vi "Sim Stripped..vi"() -> ()   [LabVIEW 2013]
doc: "This is the FPGA VI for the 10-Tap 8-Bit Camera with DRAM example. This example demonstrates how to acquire images from a 10-tap, 8-bit, extended configuration, Camera Link camera and transfer the images to the host. This example supports area scan and line scan cameras for both continuous and finite acquisitions.\n\nThis example also demonstrates the use of DRAM as a frame buffer for very high speed acquisitions. Data packing and flow-control are also employed to maximize use of the available DRAM and FIFOs in terms of both memory space and performance.\n\nAdditionally, the example demonstrates the serial server, which allows third-party camera configuration utilities to communicate with the camera using the Camera Link serial interface while this VI is running."
uses:
  <vilib>/rvi/DataTransferAndStorage/Container/XNode/niFpgaContainer.xnode
  <vilib>/Platform/TimedLoop/XDataNode/XDataNode.xnode
  <vilib>/Platform/TimedLoop/XDataNode/timing_clust.ctl
  <vilib>/Platform/TimedLoop/XDataNode/XDNodeRunTimeDep.lvlib
  <vilib>/Platform/TimedLoop/XDataNode/wakeup.ctl
  <vilib>/Platform/TimedLoop/XDataNode/nitl_modes.ctl
  <vilib>/eio/EIONode/EIONode.xnode
  <vilib>/rvi/eio/common/nirviEmuTemplateMethod_errors.vi
  <vilib>/rvi/FIFO/Fifo_Resource/nirvififoEmulationGetNumberOfElementsToRead.vi
  <vilib>/rvi/interface/RandomDataEmulation/nirviRandomDataFpgaReadWriteTemplate.vi
  <vilib>/rvi/FIFO/Fifo_Resource/nirvififoEmulationRead.vi
  <vilib>/rvi/FIFO/Fifo_Resource/nirvififoEmulationWrite.vi
  Common/CL Data to Pixels/10 Tap 8-Bit.vi
  FPGA/10-Tap Data/10-Tap Conversion Enum.ctl
  FPGA/Globals/Accumulated Sector Intensity.vi
  FPGA/Globals/Pixel Location Global.vi
  FPGA/Globals/Wing Square Wave Frequency Global.vi
  <vilib>/rvi/FIFO/Fifo_Resource/nirvififoEmulationGetNumberOfElementsToWrite.vi
  FPGA/Globals/Sector Parameter Global.vi
  Common/CL Signal Mapping.ctl
  Common/CL Configuration.ctl
  FPGA/Sector/Accumulate/Sector Parameter Cluster.ctl
panel:
  in  "[Average BG Intensity]":u8[](array[numeric])=[0, 0, 0, 0, 0, 0, 0, 0, 0, 0, 0, 0, 0, 0, 0, 0, 0, 0, 0, 0, 0, 0, 0, 0, 0, 0, 0, 0, 0, 0, 0, 0]
  in  "Sector Threshold":u8
  in  "# of Frames to Average":u8
  in  "Sector Parameters Right":T1={"Start Angle"=0.13543701171875, "End Angle"=0.30462646484375, "Inner Radius"=309, "Outter Radius"=405, "Hinge X"=1106, "Hinge Y"=803, "NumWingSectors"=8}
  in  "Sector Parameters Left":T1={"Start Angle"=0.6541748046875, "End Angle"=0.856201171875, "Inner Radius"=309, "Outter Radius"=405, "Hinge X"=947, "Hinge Y"=829, "NumWingSectors"=8}
  in  "CL Config.Configuration":T2=enum."Full"
  in  "CL Config.Signal Mapping":T3=enum."Basler 10-tap"
  in  "CL Config.Line Scan":bool
  in  "CL Config.DVAL Active High":bool=TRUE
  in  "CL Config.LVAL Active High":bool=TRUE
  in  "CL Config.FVAL Active High":bool=TRUE
  in  "CL Config.Spare Active High":bool=TRUE
  in  "Acq Control.Line Scan Height":u32
  in  "Acq Control.Frames To Acq":u32
  in  "Acq Control.Acquire":bool
  in  "Acq Control.Cancel Acq":bool
  in  "Acq Control.Ignore DVAL":bool
  in  "Acq Control.Initialize":bool
  out "Acq Status.Acq In Progress":bool
  out "Acq Status.Clocks Per Line":u32
  out "Acq Status.Frames Acq'd":u32
  out "Acq Status.Lines Per Frame":u32
  out "Acq Status.DMA Write Timeout":bool
  out "Acq Status.Initialized":bool
  in  "UART.Baud Rate":u8
  in  "UART.Transmit":bool
  in  "UART.Tx Data":u8[](array[numeric])=[0, 0, 0, 0, 0, 0, 0, 0, 0, 0] format="%02x"
  in  "UART.Set Baud Rate":bool
  in  "UART.Byte Mode":bool=TRUE
  out "UART.Rx Ready":bool
  out "UART.Break Indicator":bool
  out "UART.Framing Error":bool
  out "UART.Overrun Error":bool
  out "UART.Tx Ready":bool
  out "UART.Rx Data":u8 format="%02x"
  in  "UART.Receive":bool
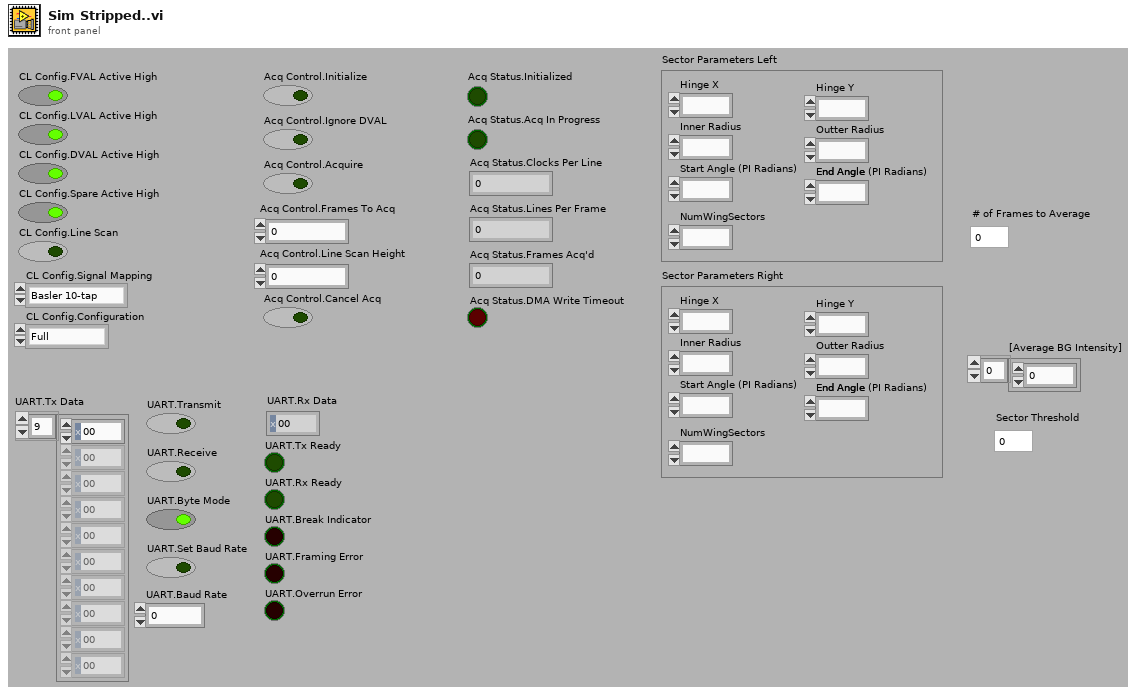
[diagram p1: front panel]
types:
  T1 = typedef "Sector Parameter Cluster.ctl" = cluster{"Start Angle":fxp<+/-,17,2>, "End Angle":fxp<+,17,3>, "Inner Radius":u16, "Outter Radius":u16, "Hinge X":u16, "Hinge Y":u16, "NumWingSectors":u8}
  T2 = typedef "CL Configuration.ctl" = enum8{"Base", "Medium", "Full"}
  T3 = typedef "CL Signal Mapping.ctl" = enum8{"Standard", "Basler 10-tap", "Vosskühler 10-tap"}
  T4 = typedef "XDNodeRunTimeDep.lvlib/timing_clust.ctl" = cluster{"Expected End [f-1]":u64, "Actual End [f-1]":u64, "Finished Late? [f-1]":bool, "Expected End [i-1]":u64, "Actual End [i-1]":u64, "Finished Late? [i-1]":bool, "Expected Start [i]":u64, "Actual Start [i]":u64, "Expected Start [f]":u64, "Actual Start [f]":u64, "Source Name":string, "Structure Name":string, "Period":i64, "Deadline":i64, "Offset":i64, "Start":i64, "Priority":i32, "Timeout":i32, "Mode":T5, "Wakeup Reason":T6, "Error":errorcluster, "Source Type":string, "Secondary Source Type":string, "Global End Time":u64, "Global Start Time":u64, "Frame Duration":u64, "Iteration Duration":u64, "Assigned CPU":i32, "I/O Scan Engine Mode":u32}
  T5 = typedef "XDNodeRunTimeDep.lvlib/nitl_modes.ctl" = enum32{"No Change", "Process missed periods, maintain original phase", "Discard missed periods, maintain original phase", "Process missed periods, ignore original phase", "Discard missed periods, ignore original phase"}
  T6 = typedef "XDNodeRunTimeDep.lvlib/wakeup.ctl" = enum32{"Normal", "Aborted", "Asynchronous wakeup", "Timing source error", "Timed loop error", "Timeout"}
  T7 = typedef "10-Tap Conversion Enum.ctl" = enum16{"10-Tap to 16 and 64", "16 and 64 to 10-Tap"}
  T8 = cluster{"Enables Valid":bool, "Frame Valid":bool, "Line Valid":bool, "Data Valid":bool}
  T9 = typedef "10-Tap 8-bit Cluster.ctl" = cluster{"Pixel 0":u8, "Pixel 1":u8, "Pixel 2":u8, "Pixel 3":u8, "Pixel 4":u8, "Pixel 5":u8, "Pixel 6":u8, "Pixel 7":u8, "Pixel 8":u8, "Pixel 9":u8}
  T10 = cluster{"Tx Data":u8[], "Transmit":bool, "Receive":bool, "Byte Mode":bool, "Set Baud Rate":bool, "Baud Rate":u8}
  T11 = cluster{"Rx Data":u8, "Turn Off Transmit":bool, "Turn Off Receive":bool, "Turn Off Set Baud Rate":bool, "Tx Ready":bool, "Rx Ready":bool, "Break Indicator":bool, "Framing Error":bool, "Overrun Error":bool}
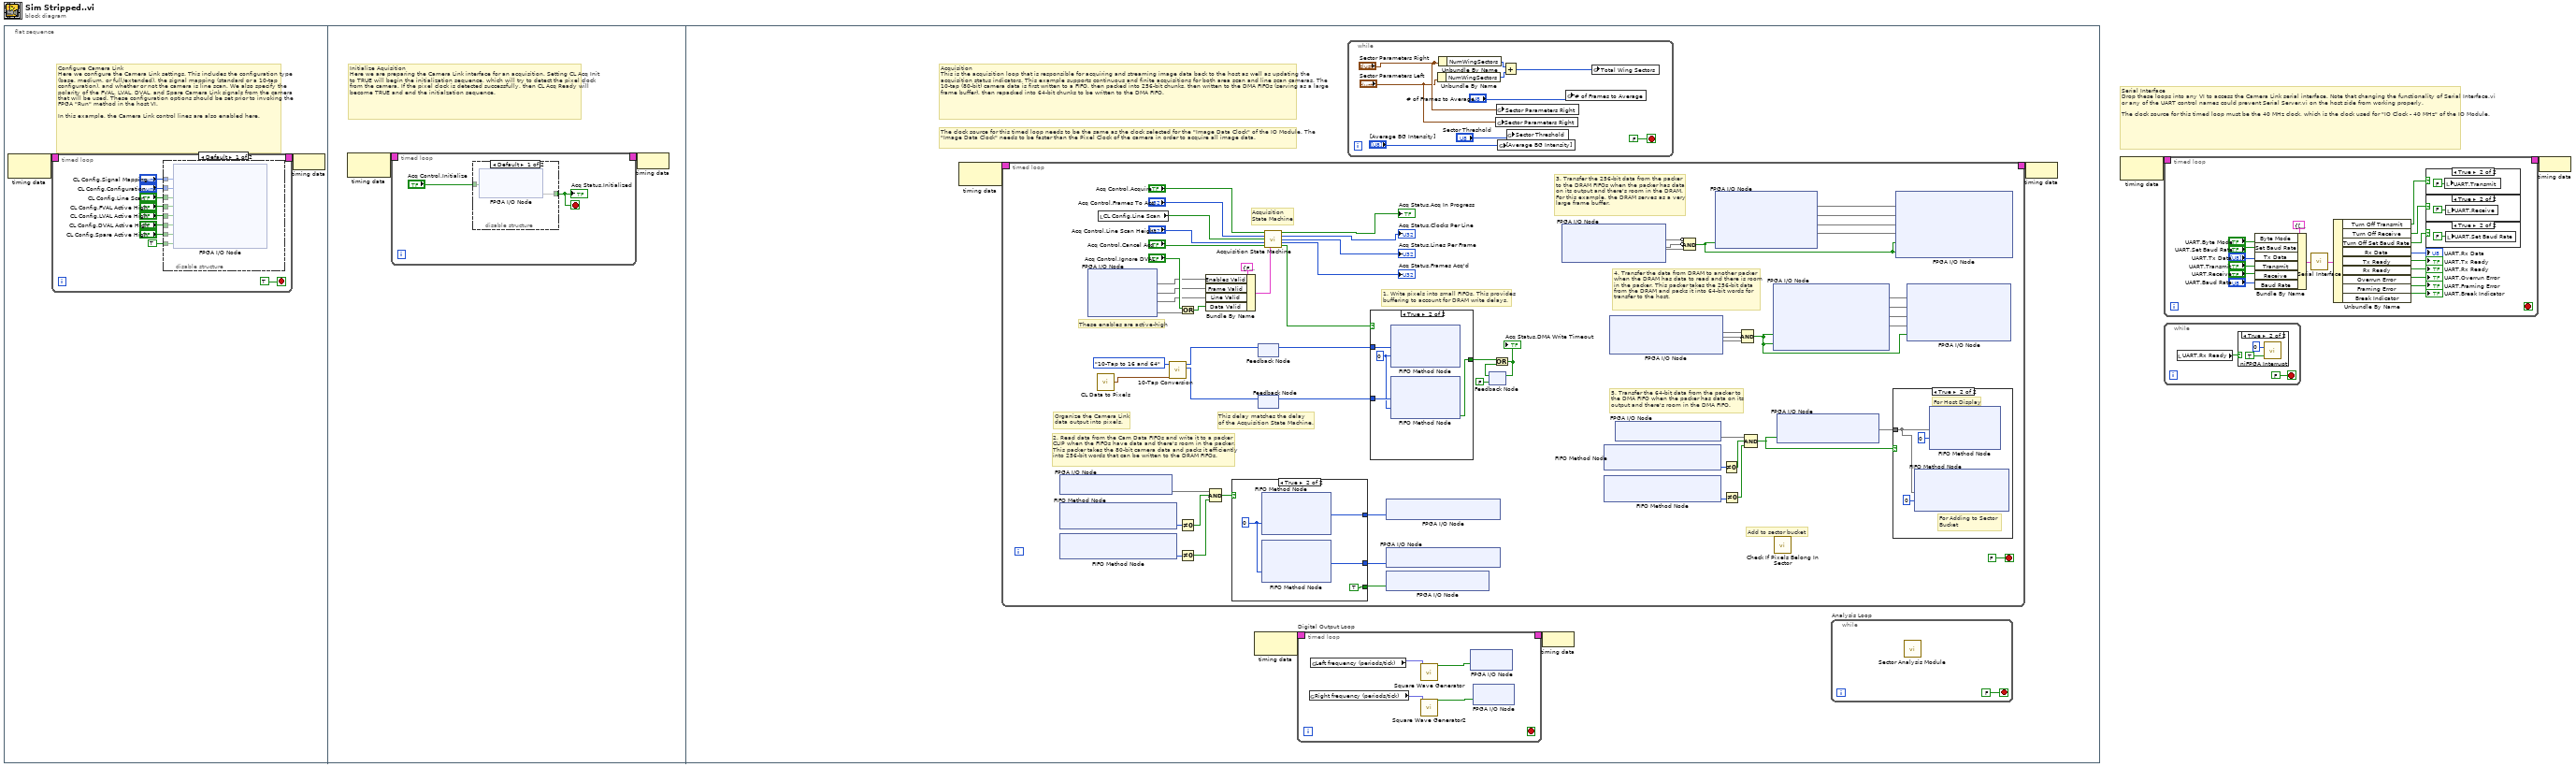
[diagram p0: block diagram]
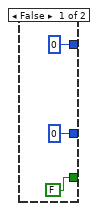
[diagram p9: hidden frame]
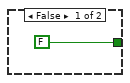
[diagram p10: hidden frame]
diagram:
  # "Serial Interface\nDrop these loops into any VI to access the Camera Link serial interface. Note that changing the functionality of Serial Interface.vi or any of the UART control names could prevent Serial Server.vi on the host side from working properly.\n\nThe clock source for this timed loop must be the 40 MHz clock, which is the clock used for \"IO Clock - 40 MHz\" of the IO Module."
  n1 = flat-sequence {
    frame #0 {
      # "Configure Camera Link\nHere we configure the Camera Link settings. This includes the configuration type (base, medium, or full/extended), the signal mapping (standard or a 10-tap configuration), and whether or not the camera is line scan. We also specify the polarity of the FVAL, LVAL, DVAL, and Spare Camera Link signals from the camera that will be used. These configuration options should be set prior to invoking the FPGA \"Run\" method in the host VI.\n\nIn this example, the Camera Link control lines are also enabled here."
      n2 = node-c288() -> (w4:T4)  [unwired: 1 in]
      n3 = timed-loop {
        timing: w4 -> [_]
        timing-out: [_] -> w3
        stop <- TRUE stop-if-true
        n4 = disable-structure shown="Default" {
          disable-tunnel: "CL Config.FVAL Active High" -> [w21 _]
          disable-tunnel: "CL Config.LVAL Active High" -> [w20 _]
          disable-tunnel: "CL Config.DVAL Active High" -> [w19 _]
          disable-tunnel: "CL Config.Spare Active High" -> [w18 _]
          disable-tunnel: "CL Config.Signal Mapping" -> [w17 _]
          disable-tunnel: "CL Config.Configuration" -> [w16 _]
          disable-tunnel: "CL Config.Line Scan" -> [w15 _]
          disable-tunnel: TRUE ("IO Module\\CL Control Enable") -> [w14 _]
          frame condition #0 {
            n5 = xnode "FPGA I/O Node"("CL Set Signal Mapping"=w17, "CL Set Configuration"=w16, "CL Set Line Scan"=w15, "CL Set FVAL Active High"=w21, "CL Set LVAL Active High"=w20, "CL Set DVAL Active High"=w19, "CL Set Spare Active High"=w18, "CL Control Enable"=w14) -> ()  [unwired: 8 in, 8 out]
          }
          frame condition #1 (active) {
          }
        }
      }
      n6 = node-c288(w3) -> ()
    }
    frame #1 {
      # "Initialize Aquisition\nHere we are preparing the Camera Link interface for an acquisition. Setting CL Acq Init to TRUE will begin the initialization sequence, which will try to detect the pixel clock from the camera. If the pixel clock is detected successfully, then CL Acq Ready will become TRUE and end the initialzation sequence."
      n7 = node-c288() -> (w27:T4)  [unwired: 1 out]
      n8 = timed-loop {
        timing: w27 -> [_]
        timing-out: [_] -> w26
        stop <- w28 stop-if-true
        n9 = disable-structure shown="Default" {
          disable-tunnel: "Acq Control.Initialize" -> [w31 w32]
          disable-tunnel: [w30 w32] -> w28
          frame condition #0 {
            n10 = xnode "FPGA I/O Node"("CL Acq Init"=w31) -> ("CL Acq Ready"=w30)  [unwired: 2 in, 2 out]
          }
          frame condition #1 (active) {
          }
        }
        "Acq Status.Initialized" <- w28
      }
      n11 = node-c288(w26) -> ()
    }
    frame #2 {
      # "The clock source for this timed loop needs to be the same as the clock selected for the \"Image Data Clock\" of the IO Module. The \"Image Data Clock\" needs to be faster than the Pixel Clock of the camera in order to acquire all image data."
      # "Acquisition\nThis is the acquisition loop that is responsible for acquiring and streaming image data back to the host as well as updating the acquisition status indicators. This example supports continuous and finite acquisitions for both area scan and line scan cameras. The 10-tap (80-bit) camera data is first written to a FIFO, then packed into 256-bit chunks, then written to the DMA FIFOs (serving as a large frame buffer), then repacked into 64-bit chunks to be written to the DMA FIFO."
      n12 = node-c288() -> (w40:T4)  [unwired: 1 in]
      n13 = timed-loop {
        timing: w40 -> [_]
        timing-out: [_] -> w39
        stop <- FALSE stop-if-true
        # "These enables are active-high"
        # "Acquisition\nState Machine"
        # "2. Read data from the Cam Data FIFOs and write it to a packer\nCLIP when the FIFOs have data and there's room in the packer.\nThis packer takes the 80-bit camera data and packs it efficiently\ninto 256-bit words that can be written to the DRAM FIFOs."
        # "Organize the Camera Link\ndata output into pixels."
        # "This delay matches the delay\nof the Acquisition State Machine."
        # "Add to sector bucket"
        # "5. Transfer the 64-bit data from the packer to\nthe DMA FIFO when the packer has data on its\noutput and there's room in the DMA FIFO."
        # "4. Transfer the data from DRAM to another packer\nwhen the DRAM has data to read and there is room\nin the packer. This packer takes the 256-bit data\nfrom the DRAM and packs it into 64-bit words for\ntransfer to the host."
        # "3. Transfer the 256-bit data from the packer\nto the DRAM FIFOs when the packer has data\non its output and there's room in the DRAM.\nFor this example, the DRAM serves as a very\nlarge frame buffer."
        # "1. Write pixels into small FIFOs. This provides\nbuffering to account for DRAM write delays."
        n14 = xnode "FPGA I/O Node"() -> ("Pack 80 to 256\\Ready For Write"=w107)  [unwired: 1 in, 1 out]
        n15 = xnode ("FIFO Method Node")() -> ("Number of Elements to Read"=w111:u32)  [unwired: 1 in, 1 out]
        n16 = xnode ("FIFO Method Node")() -> ("Number of Elements to Read"=w110:u32)  [unwired: 1 in, 1 out]
        n17 = xnode "FPGA I/O Node"() -> ("CL Output Valid"=w66, "CL Frame Valid"=w67, "CL Line Valid"=w68, "CL Data Valid"=w71)  [unwired: 4 in, 4 out]
        n18 = call-poly "CL Data to Pixels.vi"() -> ("Pixels"=w59:T9)  [unwired: 1 in]
        n19 = local read "CL Config.Line Scan"() -> (w74:bool)
        n20 = call "10-Tap Conversion.vi"("10 Tap In"=w59, "Operation"=10-Tap_Conversion_Enum."10-Tap to 16 and 64") -> ("64 Bit Out"=w60:u64, "16 Bit Out"=w61:u16)  [unwired: 7 in, 1 out]
        n21 = Or(x="Acq Control.Ignore DVAL", y=w71) -> (x .or. y?=w72:bool)
        n22 = Not Equal To 0?(x=w111) -> (x != 0?=w105:bool)
        n23 = Not Equal To 0?(x=w110) -> (x != 0?=w104:bool)
        n24 = Bundle By Name(cluster=T8 {"Enables Valid"=FALSE, "Frame Valid"=FALSE, "Line Valid"=FALSE, "Data Valid"=FALSE} ("Enables"), "Enables Valid"=w66, "Frame Valid"=w67, "Line Valid"=w68, "Data Valid"=w72) -> (w69:T8)
        n25 = Compound Arithmetic op=AND(w107, w105, w104) -> (w106:bool)
        n26 = case shown="True" w106 {
          tunnel: [u16 0 ("Element") w128] -> w112
          tunnel: [u64 0 ("Element") w127] -> w108
          tunnel: [FALSE TRUE] -> w109
          frame False {
          }
          frame True {
            w126 = 0 ("Timeout")
            n27 = xnode ("FIFO Method Node")("Timeout"=w126) -> ("Element"=w128:u16)  [unwired: 1 in, 2 out]
            n28 = xnode ("FIFO Method Node")("Timeout"=w126) -> ("Element"=w127:u64)  [unwired: 1 in, 2 out]
          }
        }
        n29 = feedback #1() -> (w113:u16)  [unwired: 1 in]
        n30 = feedback-in #1(w61) -> ()
        n31 = feedback #2() -> (w118:u64)  [unwired: 1 in]
        n32 = feedback-in #2(w60) -> ()
        n33 = call "Acquisition State Machine.vi"("Acquire"="Acq Control.Acquire", "Frames to Acquire"="Acq Control.Frames To Acq", "Line Scan"=w74, "Line Scan Height"="Acq Control.Line Scan Height", "Cancel Acq"="Acq Control.Cancel Acq", "Enables"=w69) -> ("Acq In Progress"=→"Acq Status.Acq In Progress":bool, "Num Clocks Per Line"=→"Acq Status.Clocks Per Line":u32, "Num Lines Per Frame"=→"Acq Status.Lines Per Frame":u32, "Num Frames Acq'd"=→"Acq Status.Frames Acq'd":u32, "Capture Cycle"=w102:bool)  [unwired: 4 in, 1 out]
        n34 = case shown="True" w102 {
          tunnel: [FALSE ("Timed Out?") w132] -> w116
          tunnel: w118 -> [_ w133]
          tunnel: w113 -> [_ w131]
          frame False {
          }
          frame True {
            w130 = 0 ("Timeout")
            n35 = xnode ("FIFO Method Node")("Element"=w131, "Timeout"=w130) -> ()  [unwired: 1 in, 2 out]
            n36 = xnode ("FIFO Method Node")("Element"=w133, "Timeout"=w130) -> ("Timed Out?"=w132:bool)  [unwired: 1 in, 1 out]
          }
        }
        n37 = xnode "FPGA I/O Node"("Pack 80 to 256\\Data In Upper 16"=w112) -> ()  [unwired: 1 in, 1 out]
        n38 = xnode "FPGA I/O Node"("Pack 80 to 256\\Data In Lower 64"=w108) -> ()  [unwired: 1 in, 1 out]
        n39 = xnode "FPGA I/O Node"("Pack 80 to 256\\Write Enable"=w109) -> ()  [unwired: 1 in, 1 out]
        n40 = feedback #3(FALSE) -> (w115:bool)
        n41 = Or(x=w116, y=w115) -> (x .or. y?=w114:bool)
        "Acq Status.DMA Write Timeout" <- w114
        n42 = feedback-in #3(w114) -> ()
        n43 = xnode "FPGA I/O Node"() -> ("DRAM Bank 0\\Full"=w78, "Pack 80 to 256\\Output Valid"=w97)  [unwired: 3 in, 4 out]
        n44 = xnode ("FIFO Method Node")() -> ("Number of Elements to Write"=w80:u32)  [unwired: 1 in, 1 out]
        n45 = xnode ("FIFO Method Node")() -> ("Number of Elements to Write"=w77:u32)  [unwired: 1 in, 1 out]
        n46 = xnode "FPGA I/O Node"() -> ("DRAM Bank 1\\Data_Available"=w91, "DRAM Bank 0\\Data_Available"=w89, "Pack 256 To 64\\Ready for Write"=w90)  [unwired: 3 in, 3 out]
        n47 = xnode "FPGA I/O Node"() -> ("Pack 256 To 64\\Output Valid"=w82)  [unwired: 1 in, 1 out]
        n48 = Compound Arithmetic op=AND(invert w78, invert w78, w97) -> (w92:bool)
        n49 = xnode "FPGA I/O Node"("Pack 80 to 256\\Read Enable"=w92) -> ("Pack 80 To 256\\Data Out 3"=w96, "Pack 80 To 256\\Data Out 2"=w95, "Pack 80 To 256\\Data Out 1"=w94, "Pack 80 To 256\\Data Out 0"=w93)  [unwired: 5 in, 5 out]
        n50 = Not Equal To 0?(x=w80) -> (x != 0?=w81:bool)
        n51 = Not Equal To 0?(x=w77) -> (x != 0?=w76:bool)
        n52 = Compound Arithmetic op=AND(w91, w89, w90) -> (w84:bool)
        n53 = Compound Arithmetic op=AND(w82, w81, w76) -> (w79:bool)
        n54 = xnode "FPGA I/O Node"("DRAM Bank 1\\Read"=w84, "DRAM Bank 0\\Read"=w84) -> ("DRAM Bank 1\\Read_Data_Upper"=w88, "DRAM Bank 1\\Read_Data_Lower"=w87, "DRAM Bank 0\\Read_Data_Upper"=w86, "DRAM Bank 0\\Read_Data_Lower"=w85)  [unwired: 6 in, 6 out]
        n55 = call "Check If Pixels Belong In Sector.vi"() -> ()  [unwired: 11 in, 1 out]
        n56 = xnode "FPGA I/O Node"("Pack 256 to 64\\Read Enable"=w79) -> ("Pack 256 To 64\\Data Out 64"=w83)  [unwired: 2 in, 2 out]
        n57 = case shown="True" w79 {
          tunnel: w83 -> [_ w120]
          frame False {
          }
          frame True {
            # "For Adding to Sector \nBucket"
            # "For Host Display"
            n58 = xnode ("FIFO Method Node")("Element"=w120, "Timeout"=0) -> ()  [unwired: 1 in, 2 out]
            n59 = xnode ("FIFO Method Node")("Element"=w120, "Timeout"=0) -> ()  [unwired: 1 in, 2 out]
          }
        }
        n60 = xnode "FPGA I/O Node"("DRAM Bank 1\\Write_Data_Upper"=w96, "DRAM Bank 1\\Write_Data_Lower"=w95, "DRAM Bank 0\\Write_Data_Upper"=w94, "DRAM Bank 0\\Write_Data_Lower"=w93, "DRAM Bank 1\\Write"=w92, "DRAM Bank 0\\Write"=w92) -> ()  [unwired: 6 in, 6 out]
        n61 = xnode "FPGA I/O Node"("Pack 256 To 64\\Data In 3"=w88, "Pack 256 To 64\\Data In 2"=w87, "Pack 256 To 64\\Data In 1"=w86, "Pack 256 To 64\\Data In 0"=w85, "Pack 256 to 64\\Write Enable"=w84) -> ()  [unwired: 5 in, 5 out]
      }
      n62 = node-c288() -> (w38:T4)  [unwired: 1 in]
      n63 = timed-loop "Digital Output Loop" {
        timing: w38 -> [_]
        timing-out: [_] -> w37
        stop <- _ stop-if-true
        n64 = global read "Wing Square Wave Frequency Global.vi" "Right frequency (periods/tick)"() -> (w51:fxp<+,32,0>)
        n65 = global read "Wing Square Wave Frequency Global.vi" "Left frequency (periods/tick)"() -> (w52:fxp<+,32,0>)
        n66 = call "Square Wave Generator"("frequency (periods/tick)"=w52) -> ("square wave out"=w54:bool)  [unwired: 14 in]
        n67 = call "Square Wave Generator2"("frequency (periods/tick)"=w51) -> ("square wave out"=w53:bool)  [unwired: 14 in]
        n68 = xnode "FPGA I/O Node"("TTL 0"=w54) -> ()  [unwired: 1 in, 1 out]
        n69 = xnode "FPGA I/O Node"("TTL 1"=w53) -> ()  [unwired: 1 in, 1 out]
      }
      n70 = while {
        stop <- FALSE stop-if-true
        n71 = Unbundle By Name("Sector Parameters Left") -> ("NumWingSectors"=w47:u8)
        n72 = Unbundle By Name("Sector Parameters Right") -> ("NumWingSectors"=w48:u8)
        n73 = global write "Sector Parameter Global.vi" "Sector Parameters Right"("Sector Parameters Left") -> ()
        n74 = global write "Sector Parameter Global.vi" "Sector Parameters Right"("Sector Parameters Right") -> ()
        n75 = global write "Sector Parameter Global.vi" "[Average BG Intensity]"("[Average BG Intensity]") -> ()
        n76 = Add(x=w48, y=w47) -> (x+y=w46:u8)
        n77 = global write "Sector Parameter Global.vi" "Sector Threshold"("Sector Threshold") -> ()
        n78 = global write "Pixel Location Global.vi" "# of Frames to Average"("# of Frames to Average") -> ()
        n79 = global write "Accumulated Sector Intensity.vi" "Total Wing Sectors"(w46) -> ()
      }
      n80 = node-c288(w37) -> ()
      n81 = while "Analysis Loop" {
        stop <- FALSE stop-if-true
        n82 = call "Sector Analysis Module.vi"() -> ()  [unwired: 7 in, 5 out]
      }
      n83 = node-c288(w39) -> ()
    }
  }
  n84 = node-c288() -> (w2:T4)  [unwired: 1 out]
  n85 = timed-loop {
    timing: w2 -> [_]
    timing-out: [_] -> w1
    stop <- _ stop-if-true
    n86 = Bundle By Name(cluster=T10 {"Tx Data"=[0, 0, 0, 0, 0, 0, 0, 0, 0, 0], "Transmit"=FALSE, "Receive"=FALSE, "Byte Mode"=TRUE, "Set Baud Rate"=FALSE, "Baud Rate"=0} ("UART Inputs"), "Byte Mode"="UART.Byte Mode", "Set Baud Rate"="UART.Set Baud Rate", "Tx Data"="UART.Tx Data", "Transmit"="UART.Transmit", "Receive"="UART.Receive", "Baud Rate"="UART.Baud Rate") -> (w138:T10)
    n87 = call "Serial Interface.vi"("UART Inputs"=w138) -> ("UART Outputs"=w150:T11)
    n88 = Unbundle By Name(w150) -> ("Turn Off Transmit"=w143:bool, "Turn Off Receive"=w144:bool, "Turn Off Set Baud Rate"=w140:bool, "Rx Data"=→"UART.Rx Data":u8, "Tx Ready"=→"UART.Tx Ready":bool, "Rx Ready"=→"UART.Rx Ready":bool, "Overrun Error"=→"UART.Overrun Error":bool, "Framing Error"=→"UART.Framing Error":bool, "Break Indicator"=→"UART.Break Indicator":bool)
    n89 = case shown="True" w143 {
      frame False {
      }
      frame True {
        n90 = local write "UART.Transmit"(FALSE ("UART.Transmit")) -> ()
      }
    }
    n91 = case shown="True" w144 {
      frame False {
      }
      frame True {
        n92 = local write "UART.Receive"(FALSE ("UART.Receive")) -> ()
      }
    }
    n93 = case shown="True" w140 {
      frame False {
      }
      frame True {
        n94 = local write "UART.Set Baud Rate"(FALSE ("UART.Receive")) -> ()
      }
    }
  }
  n95 = while {
    stop <- FALSE stop-if-true
    n96 = local read "UART.Rx Ready"() -> (w162:bool)
    n97 = case shown="True" w162 {
      frame False {
      }
      frame True {
        n98 = call <vilib>:"niFPGA Interrupt.vi"("Wait Until Cleared (F)"=TRUE ("Wait Until Cleared"), "IRQ Number (0)"=u8 0 ("IRQ Number")) -> ()  [unwired: 1 in]
      }
    }
  }
  n99 = node-c288(w1) -> ()
